vi "PS_SETUP_V-I-EN.vi"(0 "VISA resource name":refnum<visa-resource-name>, 1 "SEL_PS":string(combo), 11 "error in (no error)":errorcluster {"code" format="%.0x"}, 12 "Use Channel":bool[](array[boolean])=[TRUE, FALSE, FALSE, FALSE], 13 "Current Lim":sgl[](array[numeric]), 14 "Voltage Set":sgl[](array[numeric])) -> (4 "VISA resource name out":refnum<visa-resource-name>, 15 "error out":errorcluster {"code" format="%.0x"})   [LabVIEW 2018]
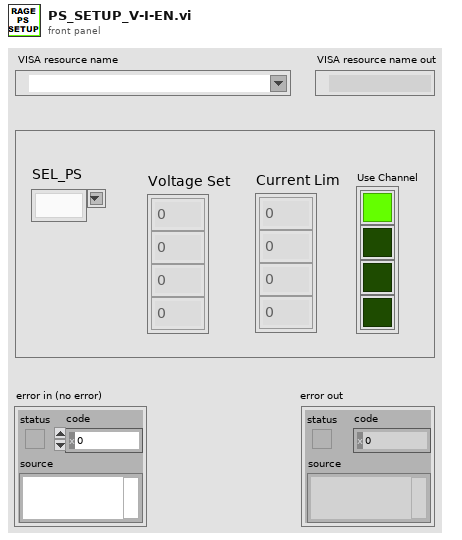
[diagram p1: front panel]
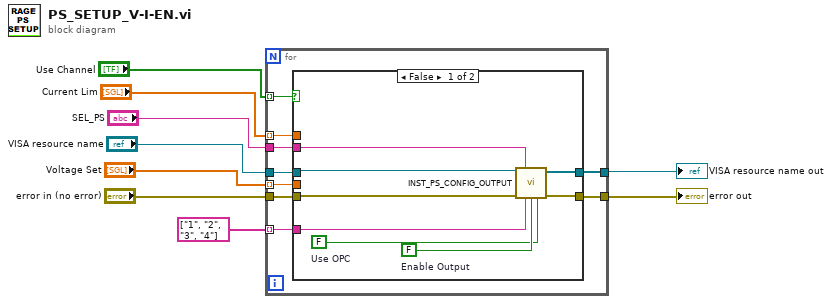
[diagram p0: block diagram]
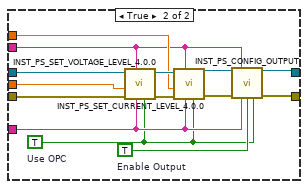
[diagram p2: hidden frame]
diagram:
  n1 = for {
    tunnel: string[] ["1", "2", "3", "4"] -> [w18] mode=indexing
    tunnel: "error in (no error)" -> [w17]
    tunnel: [w16] -> w7
    tunnel: "Use Channel" -> [w15] mode=indexing
    tunnel: "VISA resource name" -> [w14]
    tunnel: "Voltage Set" -> [w13] mode=indexing
    tunnel: [w12] -> w3
    tunnel: "SEL_PS" -> [w11]
    tunnel: "Current Lim" -> [w10] mode=indexing
    n2 = case shown="False" w15 {
      tunnel: w18 -> [w23 w29]
      tunnel: w17 -> [w19 w38]
      tunnel: [w25 w31] -> w16
      tunnel: w14 -> [w20 w39]
      tunnel: w13 -> [_ w40]
      tunnel: [w26 w33] -> w12
      tunnel: w11 -> [w24 w30]
      tunnel: w10 -> [_ w35]
      frame False {
        w22 = FALSE  # Enable Output
        w21 = FALSE  # Use OPC
        n3 = call "INST_PS_CONFIG_OUTPUT.vi"("VISA session"=w20, "SEL_PS"=w24, "error in (no error)"=w19, "Instrument Select (Output 1)"=w23, "Enable Output (False)"=w22, "Use OPC(T)"=w21) -> ("dup VISA session"=w26:refnum<visa-resource-name>, "error out"=w25:errorcluster)  [unwired: 7 in, 1 out]
      }
      frame True {
        w28 = TRUE  # Enable Output
        w27 = TRUE  # Use OPC
        n4 = call "INST_PS_SET_VOLTAGE_LEVEL_4.0.0.vi"("Use OPC(T)"=w27, "Instrument Select (Output 1)"=w29, "SEL_PS"=w30, "error in (no error)"=w38, "Voltage (0.0)"=w40, "VISA session"=w39) -> ("error out"=w37:errorcluster, "dup VISA session"=w36:refnum<visa-resource-name>)  [unwired: 4 in]
        n5 = call "INST_PS_SET_CURRENT_LEVEL_4.0.0.vi"("Use OPC(T)"=w27, "Instrument Select (Output 1)"=w29, "SEL_PS"=w30, "error in (no error)"=w37, "Current (0.0)"=w35, "VISA session"=w36) -> ("error out"=w32:errorcluster, "dup VISA session"=w34:refnum<visa-resource-name>)  [unwired: 4 in]
        n6 = call "INST_PS_CONFIG_OUTPUT.vi"("VISA session"=w34, "SEL_PS"=w30, "error in (no error)"=w32, "Instrument Select (Output 1)"=w29, "Enable Output (False)"=w28, "Use OPC(T)"=w27) -> ("dup VISA session"=w33:refnum<visa-resource-name>, "error out"=w31:errorcluster)  [unwired: 7 in, 1 out]
      }
    }
  }
  "error out" <- w7
  "VISA resource name out" <- w3
